vi "GetImage.vi"(0 "XRef":T6, 1 "State In":T3) -> (14 "Image":T2, 15 "Fatal Error Out":T1)   [LabVIEW 2021, in "FirstXNode .xnode"]
uses:
  FirstXNode .xnode
  <vilib>/XNodeSupport/XNodeXNodeRef.ctl
  State.ctl
  <vilib>/XNodeSupport/XNodeBounds.ctl
  <vilib>/XNodeSupport/XNodeInt.ctl
  <vilib>/XNodeSupport/XNodeImage.ctl
  <vilib>/XNodeSupport/XNodeErrorCluster.ctl
  <vilib>/XNodeSupport/NI_XNodeSupport.lvlib
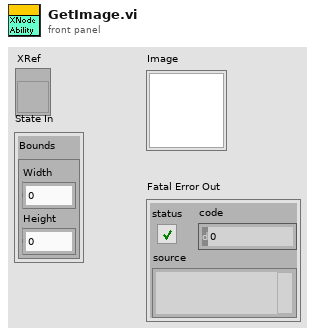
[diagram p1: front panel]
types:
  T1 = typedef "NI_XNodeSupport.lvlib/XNodeErrorCluster.ctl" = errorcluster
  T2 = typedef "NI_XNodeSupport.lvlib/XNodeImage.ctl" = picture
  T3 = typedef "FirstXNode .xnode/State.ctl" = cluster{"Bounds":T4}
  T4 = typedef "NI_XNodeSupport.lvlib/XNodeBounds.ctl" = cluster{"Width":T5, "Height":T5}
  T5 = typedef "NI_XNodeSupport.lvlib/XNodeInt.ctl" = i32
  T6 = typedef "NI_XNodeSupport.lvlib/XNodeXNodeRef.ctl" = refnum<vi>
  T7 = enum32{"Solid", "Dash", "Dot", "DashDot", "DashDotDot"}
  T8 = cluster{"Width":T5, "Style":enum32{"Solid", "Dash", "Dot", "DashDot", "DashDotDot"}}
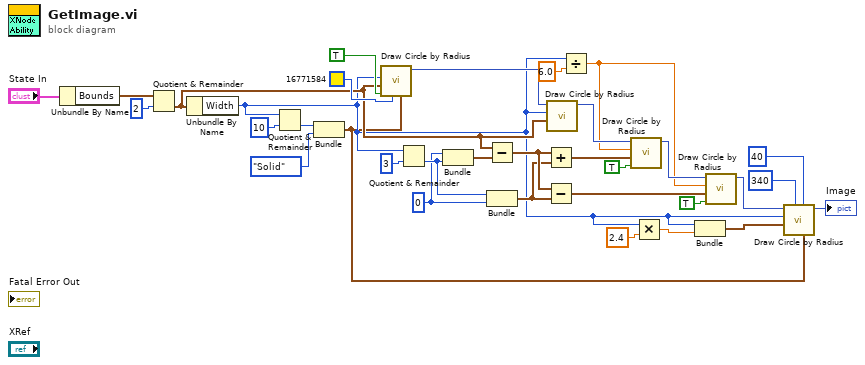
[diagram p0: block diagram]
diagram:
  w13 = i16 0 ("horizontal")
  n1 = Unbundle By Name("State In") -> ("Bounds"=w18:T4)
  n2 = Quotient & Remainder(x=w18, y=T5 2) -> (floor(x/y)=w17:T4)  [unwired: 1 out]
  n3 = Unbundle By Name(w17) -> ("Width"=w4:T5)
  n4 = Quotient & Remainder(x=w4, y=T5 10) -> (floor(x/y)=w3:T5)  [unwired: 1 out]
  n5 = Bundle("Width"=w3, "Style"=T7."Solid") -> (w1:T8)  [unwired: 1 in]
  n6 = call <vilib>:"Draw Circle by Radius.vi"("pen"=w1, "color(black)"=u32 16771584, "fill?(F)"=TRUE, "pixel center"=w17, "radius"=w4) -> ("new picture"=w31:picture)  [unwired: 6 in]
  n7 = Quotient & Remainder(x=w4, y=T5 3) -> (floor(x/y)=w14:T5)  [unwired: 1 out]
  n8 = Bundle("horizontal"=w13, "Width"=w14) -> (w15:cluster{"horizontal":i16, "Width":T5})  [unwired: 1 in]
  n9 = Subtract(x=w17, y=w15) -> (x-y=w26:T4)
  n10 = Bundle("Width"=w14, "horizontal"=w13) -> (w12:cluster{"Width":T5, "horizontal":i16})  [unwired: 1 in]
  n11 = Add(x=w26, y=w12) -> (x+y=w28:T4)
  n12 = Subtract(x=w26, y=w12) -> (x-y=w25:T4)
  n13 = call <vilib>:"Draw Circle by Radius.vi"("pixel center"=w17, "radius"=w4, "picture"=w31) -> ("new picture"=w30:picture)  [unwired: 8 in]
  n14 = Divide(x=w4, y=6.0) -> (x/y=w6:dbl)
  n15 = call <vilib>:"Draw Circle by Radius.vi"("fill?(F)"=TRUE, "pixel center"=w28, "radius"=w6, "picture"=w30) -> ("new picture"=w27:picture)  [unwired: 7 in]
  n16 = Multiply(x=w4, y=2.4) -> (x*y=w9:dbl)
  n17 = Bundle("Width"=w4, w9) -> (w10:cluster{"Width":T5, dbl})  [unwired: 1 in]
  n18 = call <vilib>:"Draw Circle by Radius.vi"("fill?(F)"=TRUE, "pixel center"=w25, "radius"=w6, "picture"=w27) -> ("new picture"=w21:picture)  [unwired: 7 in]
  n19 = call <vilib>:"Draw Circle by Radius.vi"("pen"=w1, "arc size(360)"=i16 40, "start angle(0)"=i16 340, "pixel center"=w10, "radius"=w4, "picture"=w21) -> ("new picture"=→"Image":picture)  [unwired: 5 in]
